vi "Read Running Internal Data.vi"(8 "error in (no error)":errorcluster, 11 "CIFCorePlugin in":refnum<class "CIFCorePlugin.lvclass">) -> (0 "error out":errorcluster, 2 "Running Internal Data":T1={"Refresh"=TRUE, "Iterations"=0, "Housekeep only"=FALSE, "Configured period (ns)"=0}, 3 "CIFCorePlugin out":refnum<class "CIFCorePlugin.lvclass">)   [LabVIEW 2021, in "CIFCorePlugin.lvclass"]
uses:
  CIFCorePlugin.lvclass
  CIFCorePlugin.lvclass/CIFCorePlugin.ctl
  Typedef/Running Internal Data.ctl
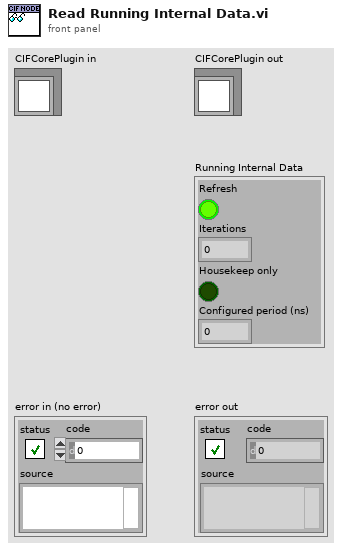
[diagram p1: front panel]
types:
  T1 = typedef "CIFCorePlugin.lvclass/Running Internal Data.ctl" = cluster{"Refresh":bool, "Iterations":i64, "Housekeep only":bool, "Configured period (ns)":i64}
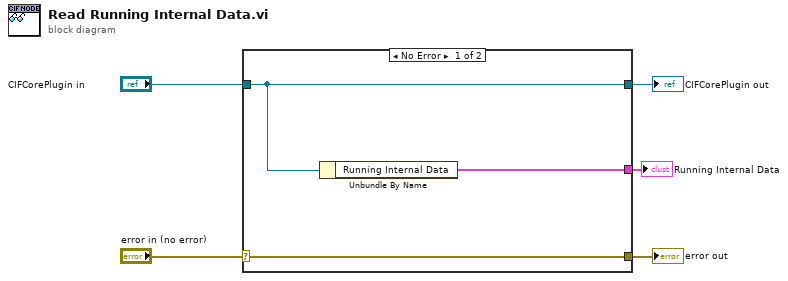
[diagram p0: block diagram]
diagram:
  n1 = case shown="No Error" "error in (no error)" {
    selector: "error in (no error)" -> [w8 w9]
    tunnel: [w8 w9] -> w4
    tunnel: [w7 w10] -> w2
    tunnel: "CIFCorePlugin in" -> [w7 w10]
    tunnel: [w6 _] -> w1
    frame No Error {
      n2 = Unbundle By Name(w7) -> ("Running Internal Data"=w6:T1)
    }
    frame Error {
    }
  }
  "error out" <- w4
  "CIFCorePlugin out" <- w2
  "Running Internal Data" <- w1
